vi "Download.vi"(6 "deadline":T1={"mode"=enum."Relative", "deadline (ms)"=30000}, 8 "error in":errorcluster, 9 "remote path":string, 10 "session in":refnum<class "Session.lvclass">, 11 "NI_SFTP.lvlib:Generic Download Controller.lvclass":refnum<class "Generic Download Controller.lvclass">) -> (0 "error out":errorcluster, 2 "session out":refnum<class "Session.lvclass">, 3 "NI_SFTP.lvlib:Generic Download Controller.lvclass 2":refnum<class "Generic Download Controller.lvclass">)   [LabVIEW 2020, in "NI_SFTP.lvlib" / "Generic Download Controller.lvclass"]
uses:
  <vilib>/net/SFTP/API/Support/Download/Generic/Generic Download Controller.lvclass
  <vilib>/net/SFTP/Session/Session.lvclass
  <vilib>/Utility/Deadline/Deadline.ctl
  <vilib>/Utility/Deadline/Mode.ctl
  <vilib>/net/SFTP/API/Support/Command/SSH_FXP_OPEN/Input.ctl
  <vilib>/net/SFTP/API/Support/Open Flags.ctl
  <vilib>/net/SFTP/API/Support/File Attributes.ctl
  <vilib>/net/SFTP/Session/Session.lvclass/Session.ctl
  <vilib>/net/SFTP/API/Support/Command/SSH_FXP_READ/Input.ctl
  <vilib>/net/SFTP/Session/Handle.ctl
  <vilib>/net/SFTP/Session/Read block size.vi
  <vilib>/net/SFTP/NI_SFTP.lvlib
  <vilib>/net/SFTP/API/Support/Command/SSH_FXP_OPEN/SSH_FXP_OPEN.lvclass
  <vilib>/net/SFTP/API/Support/Command/SSH_FXP_CLOSE/SSH_FXP_CLOSE.lvclass
  <vilib>/net/SFTP/API/Support/Command/SSH_FXP_READ/SSH_FXP_READ.lvclass
  <vilib>/Utility/Deadline/NI_Deadline.lvlib
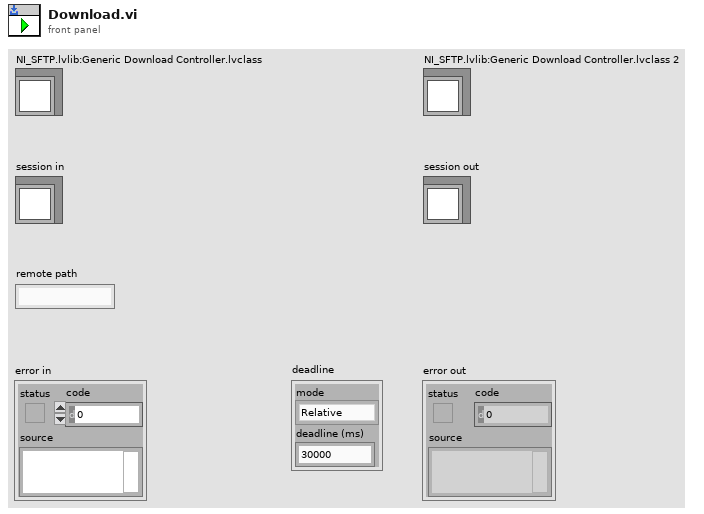
[diagram p1: front panel]
types:
  T1 = typedef "NI_Deadline.lvlib/Deadline.ctl" = cluster{"mode":T2, "deadline (ms)":u32}
  T2 = typedef "NI_Deadline.lvlib/Mode.ctl" = enum16{"Relative", "Use deadline", "Wait forever", "Nonblocking", "N/A"}
  T3 = typedef "NI_SFTP.lvlib/SSH_FXP_OPEN.lvclass/Input.ctl" = cluster{"filename":string, "open flags":T4, "file attributes":T5}
  T4 = typedef "NI_SFTP.lvlib/SSH_FXP_OPEN.lvclass/Open Flags.ctl" = cluster{"SSH_FXF_READ":bool, "SSH_FXF_WRITE":bool, "SSH_FXF_APPEND":bool, "SSH_FXF_CREAT":bool, "SSH_FXF_TRUNC":bool, "SSH_FXF_EXCL":bool}
  T5 = typedef "NI_SFTP.lvlib/File Attributes.ctl" = cluster{"SSH_FILEXFER_ATTR_SIZE":bool, "size":u64, "SSH_FILEXFER_ATTR_UIDGID":bool, "uid":u32, "gid":u32, "SSH_FILEXFER_ATTR_PERMISSIONS":bool, "permissions":u32, "SSH_FILEXFER_ATTR_ACMODTIME":bool, "atime":u32, "mtime":u32, "extended":map{string, string}}
  T6 = typedef "NI_SFTP.lvlib/SSH_FXP_READ.lvclass/Input.ctl" = cluster{"handle":T7, "offset":u64, "length":u32}
  T7 = typedef "NI_SFTP.lvlib/Session.lvclass/Handle.ctl" = u8[]
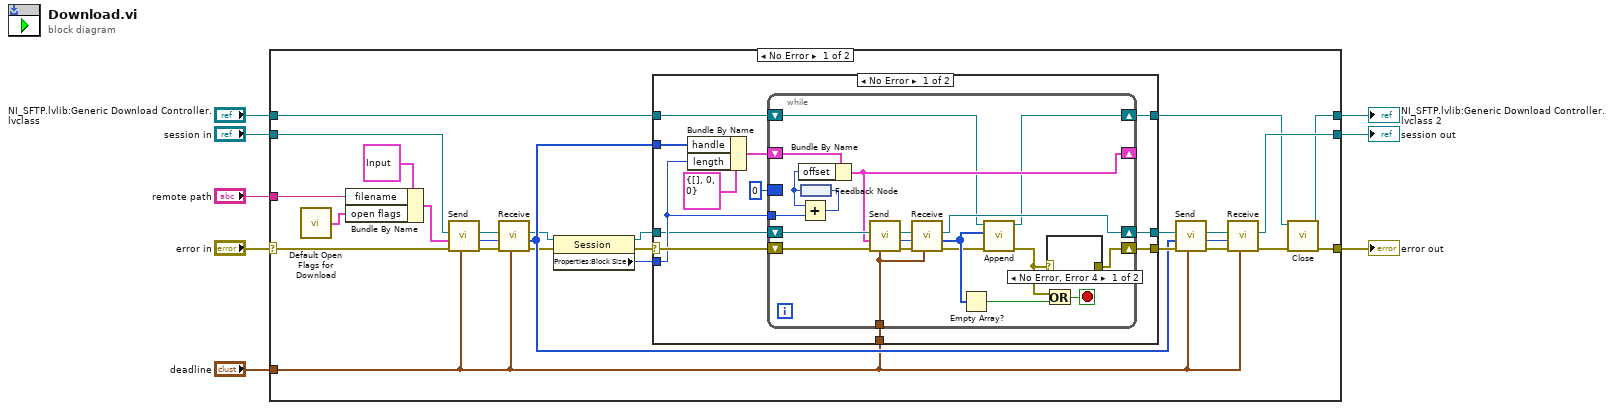
[diagram p0: block diagram]
diagram:
  n1 = case shown="No Error" "error in" {
    selector: "error in" -> [w31 w73]
    tunnel: "session in" -> [w23 w74]
    tunnel: [w30 w74] -> w7
    tunnel: [w15 w73] -> w6
    tunnel: "remote path" -> [w26 _]
    tunnel: "deadline" -> [w19 _]
    tunnel: "NI_SFTP.lvlib:Generic Download Controller.lvclass" -> [w18 w72]
    tunnel: [w14 w72] -> w1
    frame No Error {
      n2 = call <vilib>:"Default Open Flags for Download.vi"() -> ("open flags"=w25:T4)
      n3 = Bundle By Name(cluster=T3 {"filename"="", "open flags"={"SSH_FXF_READ"=FALSE, "SSH_FXF_WRITE"=FALSE, "SSH_FXF_APPEND"=FALSE, "SSH_FXF_CREAT"=FALSE, "SSH_FXF_TRUNC"=FALSE, "SSH_FXF_EXCL"=FALSE}, "file attributes"={"SSH_FILEXFER_ATTR_SIZE"=FALSE, "size"=0, "SSH_FILEXFER_ATTR_UIDGID"=FALSE, "uid"=0, "gid"=0, "SSH_FILEXFER_ATTR_PERMISSIONS"=FALSE, "permissions"=0, "SSH_FILEXFER_ATTR_ACMODTIME"=FALSE, "atime"=0, "mtime"=0, "extended"={}}} ("input"), "filename"=w26, "open flags"=w25) -> (w24:T3)
      n4 = call <vilib>:"Send.vi"("deadline"=w19, "error in"=w31, "input"=w24, "session in"=w23) -> ("error out"=w35:errorcluster, "request id"=w22:u32, "session out"=w34:refnum<class "Session.lvclass">)  [unwired: 4 in, 1 out]
      n5 = call <vilib>:"Receive.vi"("deadline"=w19, "error in"=w35, "request id"=w22, "session in"=w34) -> ("error out"=w11:errorcluster, "handle"=w20:T7, "session out"=w13:refnum<class "Session.lvclass">)  [unwired: 4 in, 1 out]
      n6 = property class="Session"(reference=w13, error in=w11) -> (reference out=w12:refnum<class "Session.lvclass">, error out=w10:errorcluster, "Properties:Block Size"=w9:i32)
      n7 = case shown="No Error" w10 {
        selector: w10 -> [w44 w71]
        tunnel: [w47 w70] -> w21
        tunnel: w12 -> [w36 w70]
        tunnel: [w46 w71] -> w32
        tunnel: w19 -> [w45 _]
        tunnel: w20 -> [w42 _]
        tunnel: w18 -> [w39 w69]
        tunnel: [w38 w69] -> w17
        tunnel: w9 -> [w37 _]
        frame No Error {
          n8 = Bundle By Name(cluster=T6 {"handle"=[], "offset"=0, "length"=0} ("input"), "handle"=w42, "length"=w37) -> (w41:T6)
          n9 = while {
            shift-right: [w58] -> w46
            shift-left: w44 -> [w65]
            shift-right: [w61] -> w47
            shift-left: w36 -> [w56]
            border: u64 0 ("len") -> [_]
            tunnel: w45 -> [w60]
            shift-right: [w54] -> _
            shift-left: w41 -> [w57]
            tunnel: w37 -> [w55]
            shift-right: [w50] -> w38
            shift-left: w39 -> [w52]
            stop <- w66 stop-if-true
            n10 = feedback #1() -> (w53:u64)
            n11 = Bundle By Name(cluster=w57, "offset"=w53) -> (w54:T6)
            n12 = Add(x=w53, y=w55) -> (x+y=w67:u64)
            n13 = feedback-in #1(w67) -> ()
            n14 = call <vilib>:"Send.vi"("deadline"=w60, "error in"=w65, "input"=w54, "session in"=w56) -> ("error out"=w62:errorcluster, "request id"=w63:u32, "session out"=w64:refnum<class "Session.lvclass">)  [unwired: 4 in, 1 out]
            n15 = call <vilib>:"Receive.vi"("deadline"=w60, "error in"=w62, "request id"=w63, "session in"=w64) -> ("error out"=w49:errorcluster, "data"=w51:u8[], "session out"=w61:refnum<class "Session.lvclass">)  [unwired: 4 in, 1 out]
            n16 = Empty Array?(array=w51) -> (empty?=w59:bool)
            n17 = call-dynamic "Append.vi"("error in (no error)"=w49, "data"=w51, "Generic Download Controller in"=w52) -> ("error out"=w48:errorcluster, "Generic Download Controller out"=w50:refnum<class "Generic Download Controller.lvclass">)  [unwired: 7 in]
            n18 = Or(x=w48, y=w59) -> (x .or. y?=w66:bool)
            n19 = case shown="No Error, Error 4" w48 {
              selector: w48 -> [_ w68]
              tunnel: [_ w68] -> w58
              frame No Error {
              }
              frame Default {
              }
            }
          }
        }
        frame Error {
        }
      }
      n20 = call <vilib>:"Send.vi"("deadline"=w19, "error in"=w32, "handle"=w20, "session in"=w21) -> ("error out"=w33:errorcluster, "request id"=w29:u32, "session out"=w28:refnum<class "Session.lvclass">)  [unwired: 4 in, 1 out]
      n21 = call <vilib>:"Receive.vi"("deadline"=w19, "error in"=w33, "request id"=w29, "session in"=w28) -> ("error out"=w16:errorcluster, "session out"=w30:refnum<class "Session.lvclass">)  [unwired: 4 in, 2 out]
      n22 = call-dynamic "Close.vi"("error in (no error)"=w16, "Generic Download Controller in"=w17) -> ("error out"=w15:errorcluster, "Generic Download Controller out"=w14:refnum<class "Generic Download Controller.lvclass">)  [unwired: 8 in]
    }
    frame Error {
    }
  }
  "error out" <- w6
  "session out" <- w7
  "NI_SFTP.lvlib:Generic Download Controller.lvclass 2" <- w1
